vi "FourFlippingCoins.vi"() -> ()   [LabVIEW 2015]
uses:
  <vilib>/Analysis/NI_AALBase.lvlib
panel:
  out "Waveform Graph":i32[](graph)
  in  "Number of Trials":dbl
  out "Number of Heads":dbl
  out "Coin 4":bool
  out "Coin 3":bool
  out "Coin 2":bool
  out "Coin 1":bool
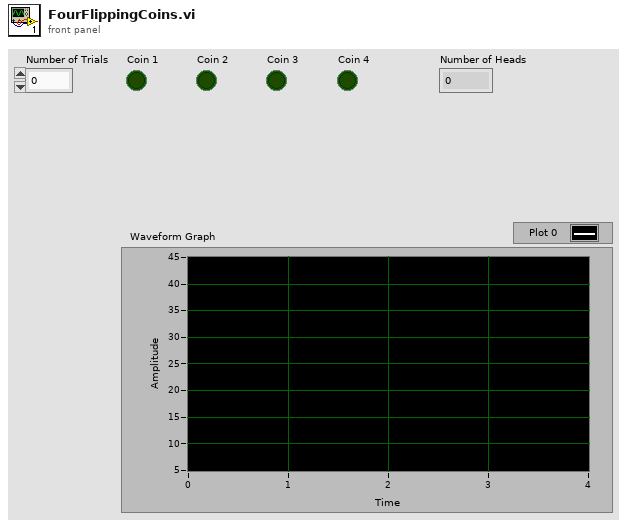
[diagram p1: front panel]
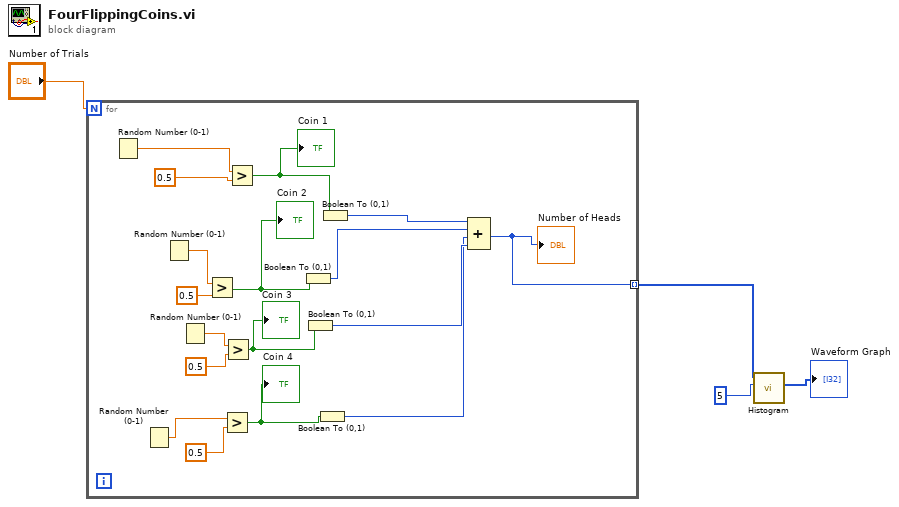
[diagram p0: block diagram]
diagram:
  n1 = for {
    N: "Number of Trials" -> [_]
    tunnel: [w5] -> w3 mode=indexing
    n2 = Random Number (0-1)() -> (number: 0 to 1=w20:dbl)
    n3 = Random Number (0-1)() -> (number: 0 to 1=w13:dbl)
    n4 = Random Number (0-1)() -> (number: 0 to 1=w17:dbl)
    n5 = Random Number (0-1)() -> (number: 0 to 1=w15:dbl)
    n6 = Greater?(x=w17, y=0.5) -> (0:w8:bool)
    "Coin 2" <- w8
    n7 = Greater?(x=w13, y=0.5) -> (0:w6:bool)
    "Coin 4" <- w6
    n8 = Greater?(x=w15, y=0.5) -> (0:w7:bool)
    "Coin 3" <- w7
    n9 = Greater?(x=w20, y=0.5) -> (0:w18:bool)
    "Coin 1" <- w18
    n10 = Boolean To (0,1)(Boolean=w8) -> (0, 1=w11:i16)
    n11 = Boolean To (0,1)(Boolean=w7) -> (0, 1=w10:i16)
    n12 = Boolean To (0,1)(Boolean=w6) -> (0, 1=w9:i16)
    n13 = Boolean To (0,1)(Boolean=w18) -> (0, 1=w21:i16)
    n14 = Compound Arithmetic op=ADD(w21, w11, w9, w10) -> (w5:i16)
    "Number of Heads" <- w5
  }
  n15 = call <vilib>:"Histogram.vi"("intervals"=5, "X"=w3) -> ("Histogram: h(x)"=→"Waveform Graph":i32[])  [unwired: 6 in, 3 out]
